vi "Analyse SUBSCRIBED.vi"(8 "Message JSON":string[](array[string]), 9 "Message Code":T1 items=["HELLO"=1, "WELCOME"=2, "ABORT"=3, "GOODBYE"=6, "ERROR"=8, "PUBLISH"=16, "PUBLISHED"=17, "SUBSCRIBE"=32, "SUBSCRIBED"=33, "UNSUBSCRIBE"=34, "UNSUBSCRIBED"=35, "EVENT"=36, "CALL"=48, "RESULT"=59, "REGISTER"=64, "REGISTERED"=65, "UNREGISTER"=66, "UNREGISTERED"=67, "INVOCATION"=68, "YIELD"=70], 10 "error in (no error)":errorcluster, 11 "reference":refnum<class "WAMP Client.lvclass">) -> (2 "error out":errorcluster, 3 "reference out":refnum<class "WAMP Client.lvclass">)   [LabVIEW 2020, in "WAMP Client.lvclass"]
uses:
  <userlib>/lvwamp/WAMP Client/WAMP Client.lvclass
  <userlib>/lvwamp/WAMP Client/TypeDef/Subscribe Result.ctl
  <userlib>/lvwamp/MessageCodes.ctl
  <userlib>/lvwamp/WAMP Client/WAMP Client.lvclass/WAMP Client.ctl
panel:
  in  "event data":T2
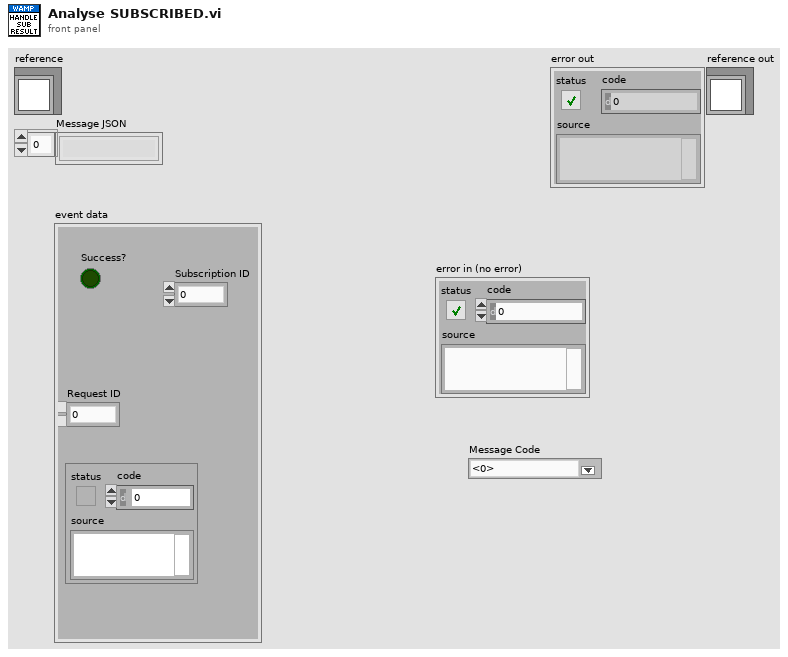
[diagram p1: front panel]
types:
  T1 = typedef "WAMP Client.lvclass/MessageCodes.ctl" = u16
  T2 = typedef "WAMP Client.lvclass/Subscribe Result.ctl" = cluster{"Success?":bool, "Error":errorcluster, "Subscription ID":dbl, "Request ID":u32}
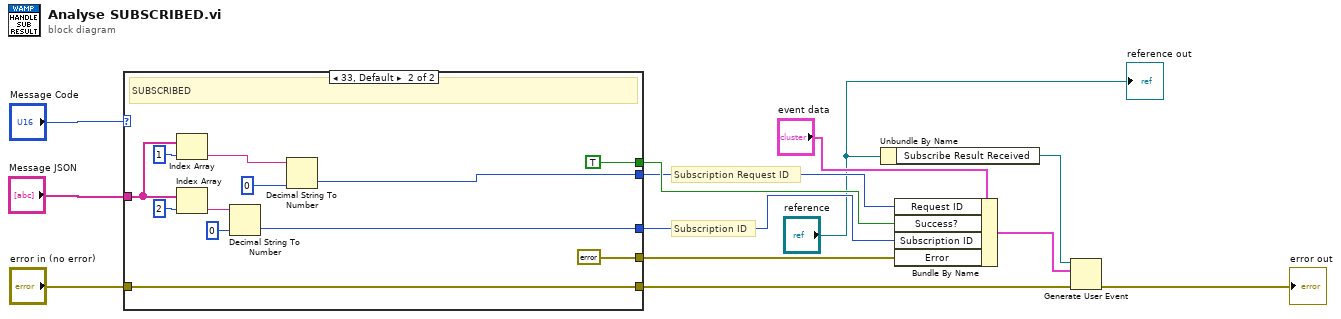
[diagram p0: block diagram]
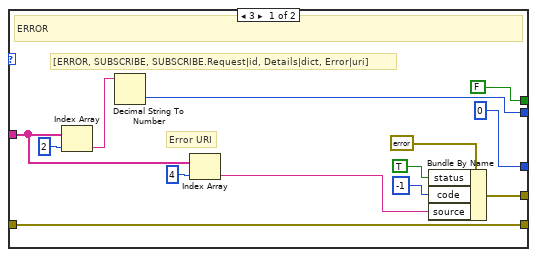
[diagram p2: hidden frame]
diagram:
  # "Subscription ID"
  # "Subscription Request ID"
  n1 = case shown="33, Default" "Message Code" {
    tunnel: "Message JSON" -> [w24 w35]
    tunnel: [w15 w28] -> w5
    tunnel: [0 w34] -> w10
    tunnel: "error in (no error)" -> [w18 w33]
    tunnel: [w18 w33] -> w3
    tunnel: [w19 errorcluster {"status"=FALSE, "code"=0, "source"=""} ("error in (no error)")] -> w8
    tunnel: [FALSE ("Success?") TRUE ("Success?")] -> w7
    frame 3 {
      # "Error URI"
      # "[ERROR, SUBSCRIBE, SUBSCRIBE.Request|id, Details|dict, Error|uri]"
      # "ERROR"
      n2 = Index Array(array=w24, index=2) -> (element=w25:string)
      n3 = Decimal String To Number(string=w25) -> (number=w15:i32)  [unwired: 2 in, 1 out]
      n4 = Index Array(array=w24, index=4) -> (element=w21:string)
      n5 = Bundle By Name(cluster=errorcluster {"status"=FALSE, "code"=0, "source"=""} ("error in (no error)"), "status"=TRUE, "code"=-1, "source"=w21) -> (w19:errorcluster)
    }
    frame 33, Default {
      # "SUBSCRIBED"
      n6 = Index Array(array=w35, index=1) -> (element=w30:string)
      n7 = Index Array(array=w35, index=2) -> (element=w37:string)
      n8 = Decimal String To Number(string=w37, default (0L)=u32 0) -> (number=w34:u32)  [unwired: 1 in, 1 out]
      n9 = Decimal String To Number(string=w30, default (0L)=u32 0) -> (number=w28:u32)  [unwired: 1 in, 1 out]
    }
  }
  n10 = Unbundle By Name("reference") -> ("Subscribe Result Received"=w6:refnum<user-event>)
  n11 = Bundle By Name(cluster="event data", "Request ID"=w5, "Success?"=w7, "Subscription ID"=w10, "Error"=w8) -> (w4:T2)
  n12 = Generate User Event(user event=w6, event data cluster=w4, error in=w3) -> (error out=→"error out":errorcluster)  [unwired: 1 in, 1 out]
  "reference out" <- "reference"
